vi "Message.vi"() -> (0 "error out":errorcluster)   [LabVIEW 2017, in "Assertion.Tests.lvlib" / "Assert False.lvlib"]
uses:
  Assert False.lvlib
  Assertion/Assertion.lvlib
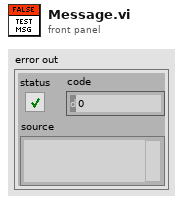
[diagram p1: front panel]
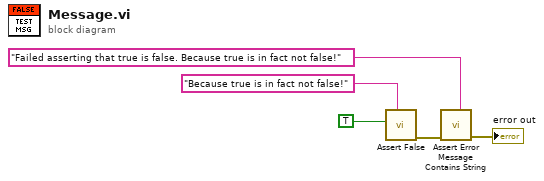
[diagram p0: block diagram]
diagram:
  n1 = call "Assert False.vi"("Message (\"\")"="Because true is in fact not false!" ("Message (\"\")"), "Condition"=TRUE) -> ("error out"=w4:errorcluster)  [unwired: 9 in]
  n2 = call "Assert Error Message Contains String.vi"("Expected"="Failed asserting that true is false. Because true is in fact not false!" ("y"), "error in (no error)"=w4) -> ("error out"=→"error out":errorcluster)  [unwired: 9 in]
